vi "Get Path to Latest Image.vi"(8 "Error In":errorcluster) -> (0 "error out":errorcluster, 3 "Path to Latest Image":string)   [LabVIEW 2014]
uses:
  Controls/Image Names in a Folder.ctl
  <vilib>/httpClient/LabVIEWHTTPClient.lvlib
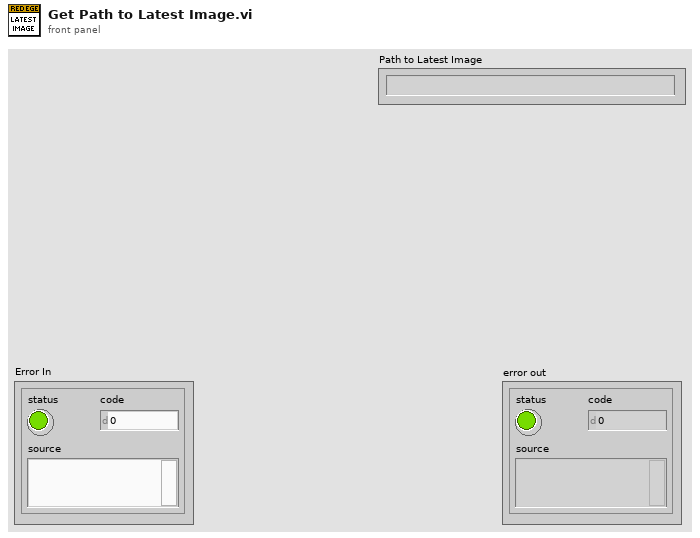
[diagram p1: front panel]
types:
  T1 = typedef "Image Names in a Folder.ctl" = cluster{"directories":string[], "files":cluster{"name":string, "size":i32}[]}
  T2 = typedef "LabVIEWHTTPClient.lvlib/ClientHandle.ctl" = refnum<k1>
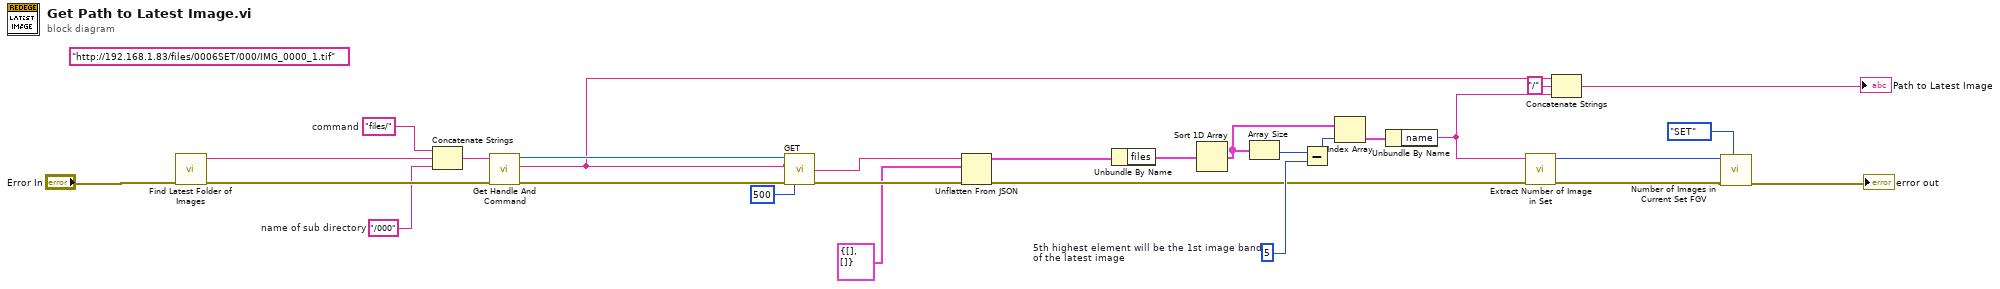
[diagram p0: block diagram]
diagram:
  w13 = 5  # 5th highest element will be the 1st image band of the latest image
  w21 = "/000"  # name of sub directory
  w25 = "files/"  # command
  (unwired) "http://192.168.1.83/files/0006SET/000/IMG_0000_1.tif" ("url")
  n1 = call "Find Latest Folder of Images.vi"("Error In"="Error In") -> ("error out"=w26:errorcluster, "Latest Folder of Images"=w24:string)  [unwired: 9 in]
  n2 = Concatenate Strings(w25, w24, w21) -> (w22:string)
  n3 = call "Get Handle And Command.vi"("Error In"=w26, "Command"=w22) -> ("Error Out"=w27:errorcluster, "Command URL"=w10:string, "RedEdge client handle out"=w28:T2)  [unwired: 6 in]
  n4 = call <vilib>:"GET.vi"("client handle"=w28, "url"=w10, "error in (no error)"=w27, "timeout (10000)"=500) -> ("body"=w20:string, "error out"=w19:errorcluster)  [unwired: 8 in, 2 out]
  n5 = Unflatten From JSON(JSON string=w20, type and defaults=T1 {"directories"=[], "files"=[]} ("Image Names in a Folder"), error in (no error)=w19) -> (value=w17:T1, error out=w5:errorcluster)  [unwired: 4 in]
  n6 = Unbundle By Name(w17) -> ("files"=w16:cluster{"name":string, "size":i32}[])
  n7 = Sort 1D Array(array=w16) -> (sorted array=w15:cluster{"name":string, "size":i32}[])
  n8 = Array Size(array=w15) -> (size(s)=w14:i32)
  n9 = Subtract(x=w14, y=w13) -> (x-y=w12:i32)
  n10 = Index Array(array=w15, index=w12) -> (element=w11:cluster{"name":string, "size":i32})
  n11 = Unbundle By Name(w11) -> ("name"=w6:string)
  n12 = call "Extract Number of Image in Set.vi"("Error In"=w5, "Image Name"=w6) -> ("Error Out"=w4:errorcluster, "Number of pics taken"=w3:i32)  [unwired: 8 in]
  n13 = Concatenate Strings(w10, "/" ("string"), w6) -> (→"Path to Latest Image":string)
  n14 = call "Number of Images in Current Set FGV.vi"("Operation"=enum16{"GET", "SET"}."SET", "Error In"=w4, "Number of pics taken"=w3) -> ("Error Out"=→"error out":errorcluster)  [unwired: 7 in, 1 out]
